vi "Sensor Queue Handler.vi"(7 "Action":T3, 8 "error in (no error)":errorcluster, 10 "Message in":T1, 11 "User event in":refnum<user-event>) -> (0 "error out":errorcluster, 1 "Event Registration Refnum":refnum<event-registration>, 2 "Timeout":i32, 3 "User event out":refnum<user-event>)   [LabVIEW 2017]
uses:
  Type Definitions/Queue FG Options.ctl
  Type Definitions/Sensor Message.ctl
  Type Definitions/Sensor States.ctl
  Type Definitions/Timer States.ctl
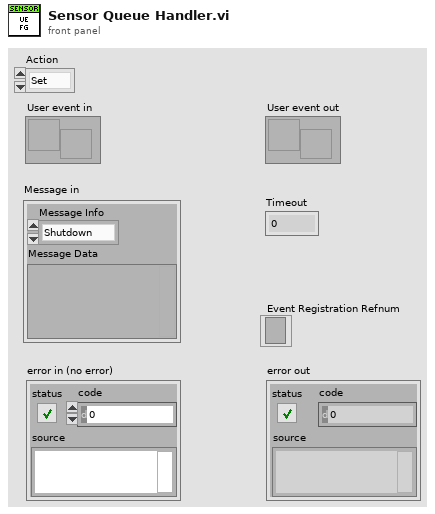
[diagram p1: front panel]
types:
  T1 = typedef "Sensor Message.ctl" = cluster{"Message Info":T2, "Message Data":variant}
  T2 = typedef "Sensor States.ctl" = enum16{"Shutdown", "Initial", "Idle"}
  T3 = typedef "Queue FG Options.ctl" = enum16{"Set", "Get", "Read", "Write", "Destroy"}
  T4 = typedef "Timer States.ctl" = enum16{"Set", "Get"}
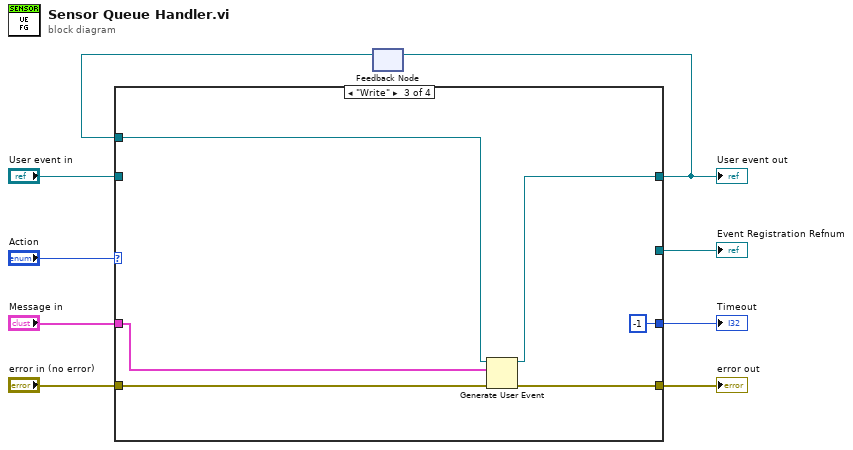
[diagram p0: block diagram]
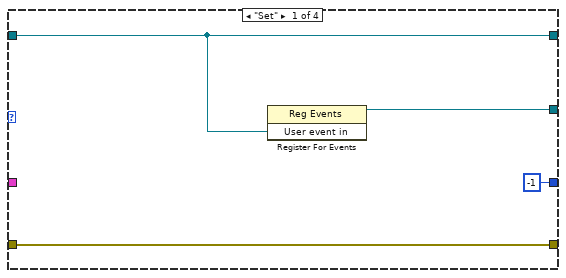
[diagram p2: hidden frame]
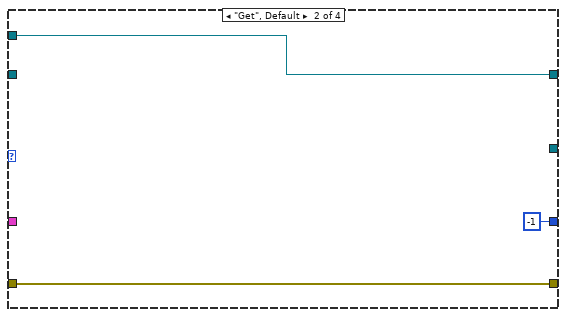
[diagram p3: hidden frame]
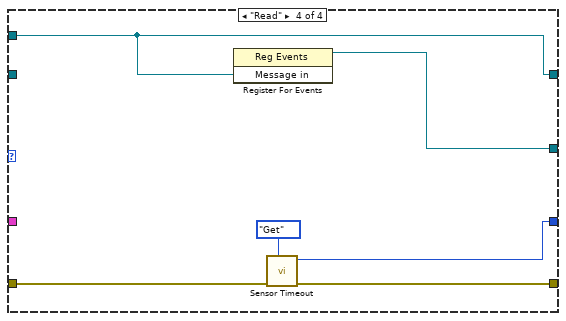
[diagram p4: hidden frame]
diagram:
  n1 = feedback #1() -> (w6:refnum<user-event>)  [unwired: 1 in]
  n2 = case shown="\"Write\"" "Action" {
    tunnel: "error in (no error)" -> [w13 w16 w22 w28]
    tunnel: [w13 w16 w21 w26] -> w7
    tunnel: w6 -> [_ w14 w18 w23]
    tunnel: "Message in" -> [_ _ w17 _]
    tunnel: "User event in" -> [w11 _ _ _]
    tunnel: [w10 _ _ w27] -> w1
    tunnel: [-1 ("Timeout") -1 ("Timeout") -1 ("Timeout") w24] -> w4
    tunnel: [w11 w14 w19 w23] -> w3
    frame "Set" {
      n3 = register-events(w11) -> (reference out=w10:refnum<event-registration>)  [unwired: 2 in, 1 out]
    }
    frame "Get", Default {
    }
    frame "Write" {
      n4 = Generate User Event(user event=w18, event data cluster=w17, error in=w22) -> (user event out=w19:refnum<user-event>, error out=w21:errorcluster)  [unwired: 1 in]
    }
    frame "Read" {
      n5 = register-events(w23) -> (reference out=w27:refnum<event-registration>)  [unwired: 2 in, 1 out]
      n6 = call "Sensor Timeout.vi"("Timer States"=Timer_States."Get", "error in (no error)"=w28) -> ("error out"=w26:errorcluster, "Timeout"=w24:i32)  [unwired: 8 in]
    }
  }
  "error out" <- w7
  "Timeout" <- w4
  "User event out" <- w3
  "Event Registration Refnum" <- w1
  n7 = feedback-in #1(w3) -> ()
